vi "CountsToUnits.vi"(7 "Units (Encoder Counts)":T1=enum."Encoder Counts", 9 "Gear Ratio":dbl, 10 "Counts/Rev":dbl, 11 "Encoder Counts":i32) -> (5 "Value in Units":dbl)   [LabVIEW 2010]
uses:
  Typedefs/Units_Enum.ctl
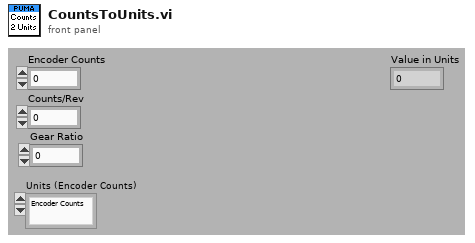
[diagram p1: front panel]
types:
  T1 = typedef "Units_Enum.ctl" = enum16{"Radians", "Encoder Counts", "Revolutions", "Degrees"}
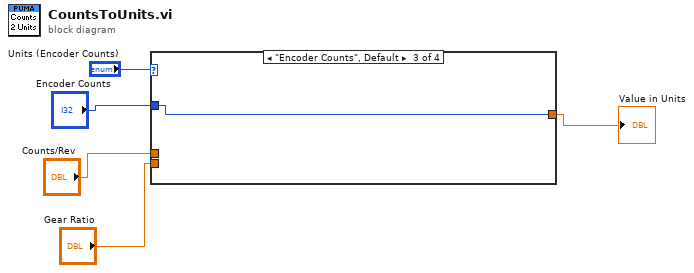
[diagram p0: block diagram]
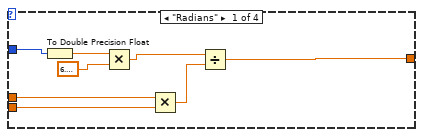
[diagram p2: hidden frame]
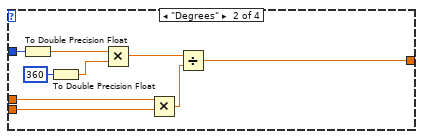
[diagram p3: hidden frame]
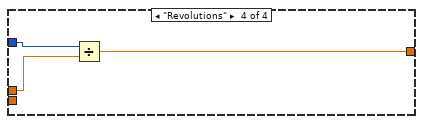
[diagram p4: hidden frame]
diagram:
  n1 = case shown="\"Encoder Counts\", Default" "Units (Encoder Counts)" {
    tunnel: "Encoder Counts" -> [w8 w22 w23 w26]
    tunnel: [w9 w18 w23 w25] -> w5
    tunnel: "Counts/Rev" -> [w7 w17 _ w24]
    tunnel: "Gear Ratio" -> [w6 w16 _ _]
    frame "Radians" {
      n2 = To Double Precision Float(number=w8) -> (double precision float=w13:dbl)
      n3 = Multiply(x=w13, y=6.283185307179586) -> (x*y=w11:dbl)
      n4 = Multiply(x=w7, y=w6) -> (x*y=w10:dbl)
      n5 = Divide(x=w11, y=w10) -> (x/y=w9:dbl)
    }
    frame "Degrees" {
      n6 = To Double Precision Float(number=w22) -> (double precision float=w21:dbl)
      n7 = To Double Precision Float(number=360) -> (double precision float=w14:dbl)
      n8 = Multiply(x=w21, y=w14) -> (x*y=w20:dbl)
      n9 = Multiply(x=w17, y=w16) -> (x*y=w19:dbl)
      n10 = Divide(x=w20, y=w19) -> (x/y=w18:dbl)
    }
    frame "Encoder Counts", Default {
    }
    frame "Revolutions" {
      n11 = Divide(x=w26, y=w24) -> (x/y=w25:dbl)
    }
  }
  "Value in Units" <- w5
